vi "Write to file.vi"(8 "error in":errorcluster, 10 "input string":string, 11 "file path":path) -> (0 "error out":errorcluster)   [LabVIEW 2024]
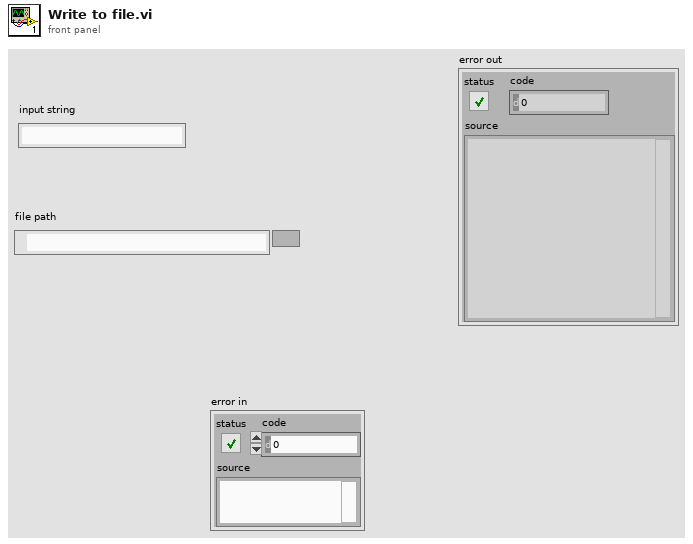
[diagram p1: front panel]
types:
  T1 = enum16{"open", "replace", "create", "open or create", "replace or create", "replace or create with confirmation"}
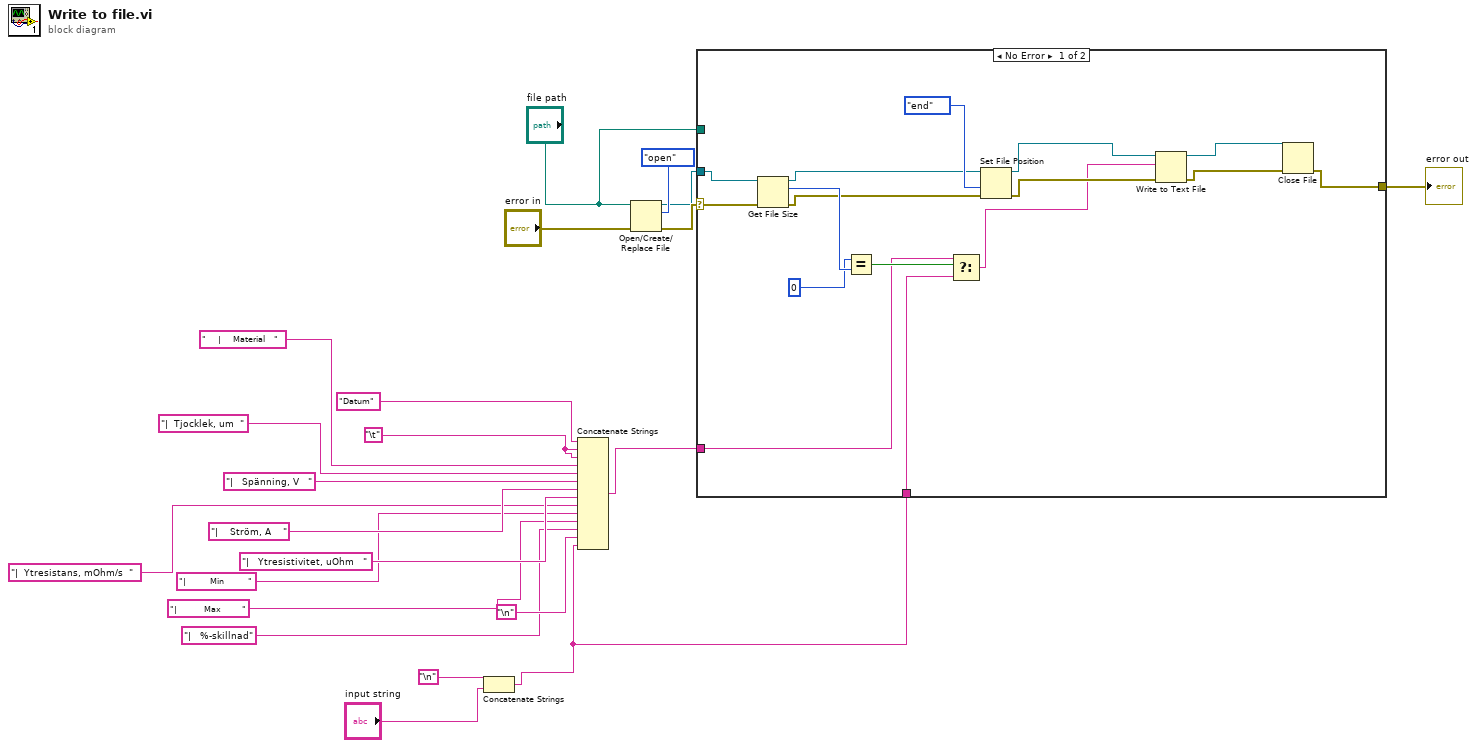
[diagram p0: block diagram]
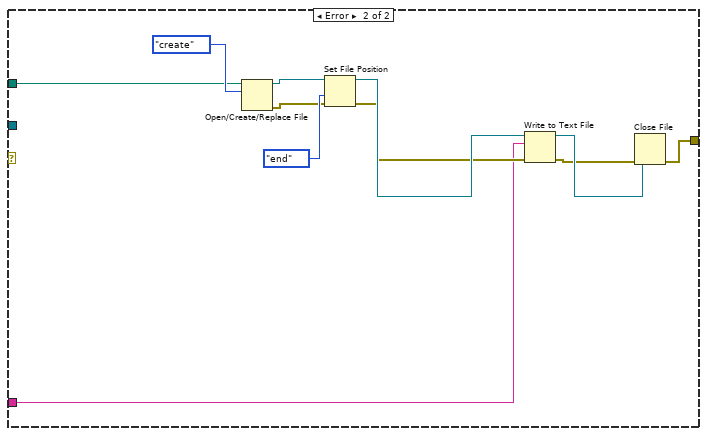
[diagram p2: hidden frame]
diagram:
  w8 = "\t"
  n1 = Concatenate Strings("\n", "input string") -> (w6:string)
  n2 = Concatenate Strings("Datum" ("string"), w8, w8, "    |    Material   " ("string"), "|  Tjocklek, um  " ("string"), "|   Spänning, V   " ("string"), "|    Ström, A    " ("string"), "|   Ytresistivitet, uOhm   " ("string"), "|  Ytresistans, mOhm/s  " ("string"), "|        Min        " ("string"), "|         Max       " ("string"), "|   %-skillnad" ("string"), "\n", w6) -> (w11:string)
  n3 = Open/Create/Replace File(file path (use dialog)="file path", error in="error in", operation (0:open)=T1."open") -> (refnum out=w16:refnum<file>, error out=w17:errorcluster)  [unwired: 3 in, 1 out]
  n4 = case shown="No Error" w17 {
    selector: w17 -> [w32 _]
    tunnel: [w33 w40] -> w21
    tunnel: w16 -> [w31 _]
    tunnel: "file path" -> [_ w43]
    tunnel: w11 -> [w25 w39]
    tunnel: w6 -> [w24 _]
    frame No Error {
      n5 = Get File Size(file=w31, error in=w32) -> (refnum out=w26:refnum<file>, size (in bytes)=w30:i64, 0:w27:errorcluster)
      n6 = Equal?(x=i64 0, y=w30) -> (x = y?=w28:bool)
      n7 = Select(t=w25, s=w28, f=w24) -> (s? t:f=w23:string)
      n8 = Set File Position(refnum=w26, from (0:start)=enum16{"start", "end", "current"}."end", error in=w27) -> (refnum out=w37:refnum<file>, error out=w36:errorcluster)  [unwired: 1 in]
      n9 = Write to Text File(file (use dialog)=w37, text=w23, error in=w36) -> (refnum out=w38:refnum<file>, error out=w35:errorcluster)  [unwired: 1 in, 1 out]
      n10 = Close File(refnum=w38, error in=w35) -> (error out=w33:errorcluster)  [unwired: 1 out]
    }
    frame Error {
      n11 = Open/Create/Replace File(file path (use dialog)=w43, operation (0:open)=T1."create") -> (refnum out=w41:refnum<file>, error out=w42:errorcluster)  [unwired: 4 in, 1 out]
      n12 = Set File Position(refnum=w41, from (0:start)=enum16{"start", "end", "current"}."end", error in=w42) -> (refnum out=w48:refnum<file>, error out=w47:errorcluster)  [unwired: 1 in]
      n13 = Write to Text File(file (use dialog)=w48, text=w39, error in=w47) -> (refnum out=w49:refnum<file>, error out=w46:errorcluster)  [unwired: 1 in, 1 out]
      n14 = Close File(refnum=w49, error in=w46) -> (error out=w40:errorcluster)  [unwired: 1 out]
    }
  }
  "error out" <- w21
